vi "Serialize - JSON.vi"(8 "error in (no error)":errorcluster, 11 "Single_Array in":refnum<class "Single_Array.lvclass">) -> (0 "error out":errorcluster, 2 "Serialized JSON":string, 3 "Single_Array out":refnum<class "Single_Array.lvclass">)   [LabVIEW 2016, in "Base Data Class.lvlib" / "Single_Array.lvclass"]
uses:
  Single_Array.lvclass
  G:/sw_repo/For Builds/Reusable/Data/Data.lvclass
  Data.lvclass/Data.ctl
  Single_Array.lvclass/Single_Array.ctl
  Read Data ID.vi
  Data.lvclass
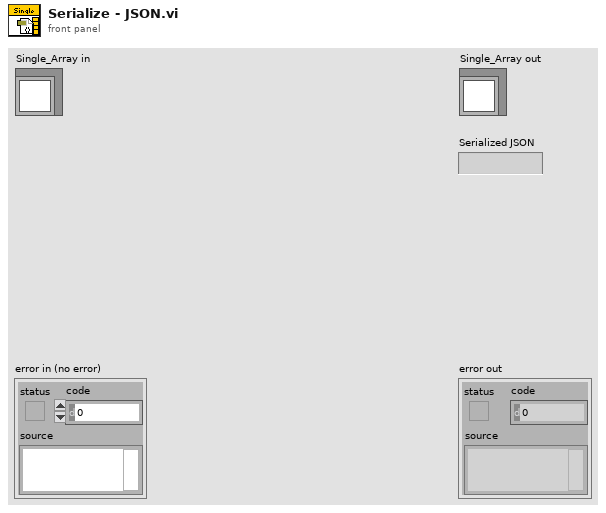
[diagram p1: front panel]
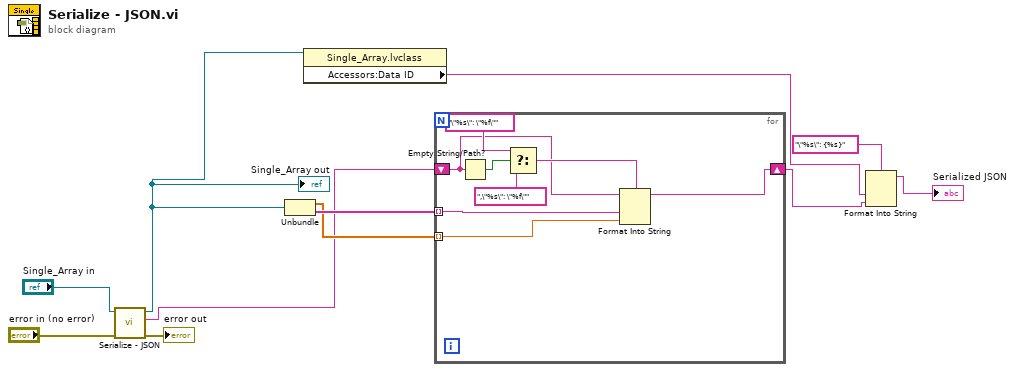
[diagram p0: block diagram]
diagram:
  n1 = call-parent "Serialize - JSON.vi"("error in"="error in (no error)", "Data in"="Single_Array in") -> ("error out"=→"error out":errorcluster, "Serialized JSON"=w6:string, "Data out"=w3:refnum<class "Single_Array.lvclass">)  [unwired: 7 in]
  "Single_Array out" <- w3
  n2 = Unbundle(w3) -> (w7:sgl[], w8:string[])
  n3 = property class="Single_Array.lvclass"(reference=w3) -> ("Accessors:Data ID"=w2:string)  [unwired: 1 in, 2 out]
  n4 = for {
    tunnel: w8 -> [w19] mode=indexing
    tunnel: w7 -> [w18] mode=indexing
    shift-right: [w12] -> w4
    shift-left: w6 -> [w13]
    n5 = Empty String/Path?(string/path=w13) -> (empty?=w17:bool)
    n6 = Select(t="\"%s\": \"%f\"" ("format string"), s=w17, f=",\"%s\": \"%f\"" ("format string")) -> (s? t:f=w14:string)
    n7 = Format Into String(format string=w14, initial string=w13, w19, w18) -> (resulting string=w12:string)  [unwired: 1 in, 1 out]
  }
  n8 = Format Into String(format string="\"%s\": {%s}", w2, w4) -> (resulting string=→"Serialized JSON":string)  [unwired: 2 in, 1 out]
